vi "get_moving_statuses.vi"(8 "error in (no error)":errorcluster caption="错误输入（无错误）", 11 "MotorSystem输入":refnum<class "MotorSystem.lvclass">) -> (0 "error out":errorcluster caption="错误输出", 2 "moving?":bool[](array[boolean]), 3 "MotorSystem输出":refnum<class "MotorSystem.lvclass">)   [LabVIEW 2016, in "MotionControl.lvlib" / "MotorSystem.lvclass"]
uses:
  <userlib>/MotionControl/MotorSystem/MotorSystem.lvclass
  <userlib>/MotionControl/MotorSystem/MotorSystem.lvclass/MotorSystem.ctl
  <userlib>/MotionControl/OneMotion/OneMotion.lvclass
  <userlib>/MotionControl/StepMotor/StepMotor.lvclass
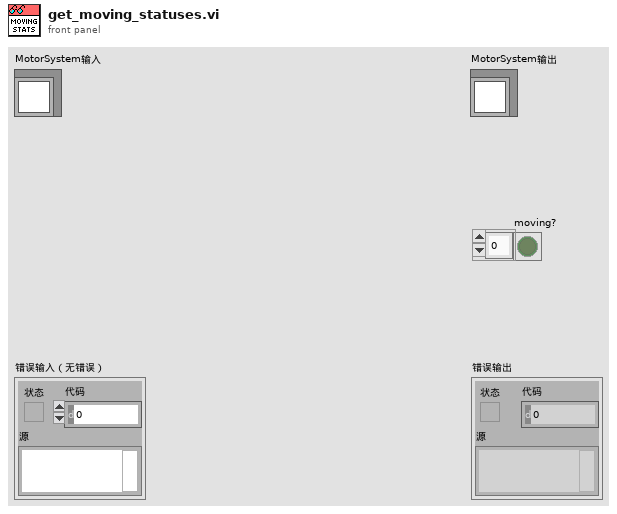
[diagram p1: front panel]
types:
  T1 = typedef "MotionControl.lvlib/MotorSystem.lvclass/MotionCluster.ctl" = cluster{"OneMotion.lvclass":refnum<class "OneMotion.lvclass">, "connected?":bool, "default enabled?":bool, "enabled?":bool}
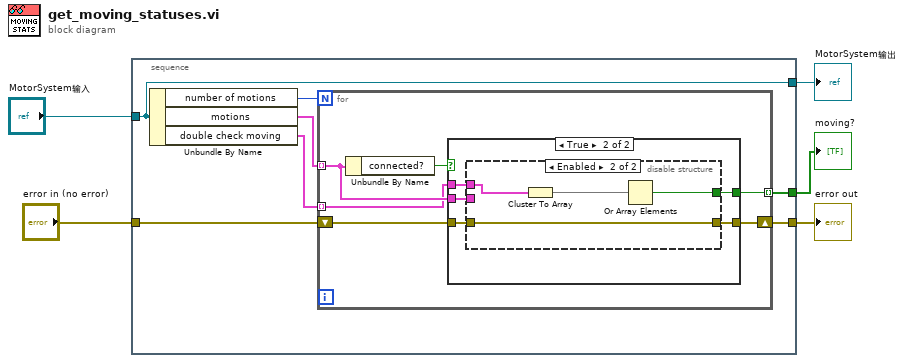
[diagram p0: block diagram]
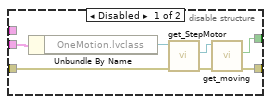
[diagram p3: hidden frame]
diagram:
  n1 = stacked-sequence {
    tunnel: [w12] -> w5
    tunnel: "MotorSystem输入" -> [w10]
    tunnel: "error in (no error)" -> [w8]
    tunnel: [w11] -> w1
    tunnel: [w10] -> w2
    frame #0 {
      n2 = Unbundle By Name(w10) -> ("number of motions"=w6:i32, "motions"=w9:T1[], "double check moving"=w7:cluster{"1st check":bool, "2nd check":bool}[])
      n3 = for {
        N: w6 -> [_]
        tunnel: [w17] -> w11 mode=indexing
        tunnel: w9 -> [w15] mode=indexing
        shift-right: [w18] -> w12
        shift-left: w8 -> [w16]
        tunnel: w7 -> [w13] mode=indexing
        n4 = Unbundle By Name(w15) -> ("connected?"=w14:bool)
        n5 = case shown="True" w14 {
          tunnel: [w19 w24] -> w18
          tunnel: [_ w23] -> w17
          tunnel: w15 -> [_ w22]
          tunnel: w16 -> [w19 w21]
          tunnel: w13 -> [_ w20]
          frame False {
          }
          frame True {
            n6 = disable-structure shown="Enabled" {
              disable-tunnel: [w28 w35] -> w24
              disable-tunnel: [w27 w32] -> w23
              disable-tunnel: w22 -> [w26 _]
              disable-tunnel: w21 -> [w25 w35]
              disable-tunnel: w20 -> [_ w34]
              frame Disabled {
                n7 = Unbundle By Name(w26) -> ("OneMotion.lvclass"=w31:refnum<class "OneMotion.lvclass">)
                n8 = call <userlib>:"get_StepMotor.vi"("error in (no error)"=w25, "OneMotion输入"=w31) -> ("error out"=w29:errorcluster, "StepMotor.lvclass"=w30:refnum<class "StepMotor.lvclass">)  [unwired: 7 in, 1 out]
                n9 = call <userlib>:"get_moving.vi"("error in (no error)"=w29, "StepMotor输入"=w30) -> ("error out"=w28:errorcluster, "moving?"=w27:bool)  [unwired: 7 in, 1 out]
              }
              frame Enabled {
                n10 = Cluster To Array(cluster=w34) -> (array=w33:bool[])
                n11 = Or Array Elements(Boolean array=w33) -> (logical OR=w32:bool)
              }
            }
          }
        }
      }
    }
  }
  "error out" <- w5
  "MotorSystem输出" <- w2
  "moving?" <- w1
